vi "InitiateMultiPoint.vi"(8 "error in (no error)":errorcluster, 11 "HP3458aDMM in":refnum<class "HP3458aDMM.lvclass">) -> (0 "error out":errorcluster, 3 "HP3458aDMM out":refnum<class "HP3458aDMM.lvclass">)   [LabVIEW 2014, in "SamplerPlugins.lvlib" / "HP3458aDMM.lvclass"]
uses:
  HP3458aDMM.lvclass
  <instrlib>/Agilent 3458/Agilent 3458.lvlib
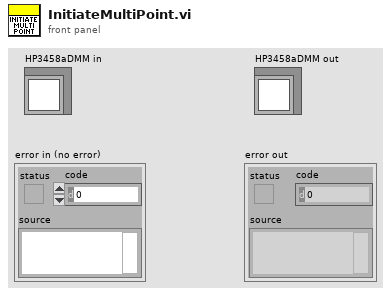
[diagram p1: front panel]
types:
  T1 = typedef "SamplerPlugins.lvlib/SamplerPluginsBase.lvclass/ConfigMultiPointParams.ctl" = cluster{"iTriggerCount":i32, "iSampleCount":i32, "eSampleClock":u16, "dSampleInterval":dbl}
  T2 = typedef "SamplerPlugins.lvlib/SamplerPluginsBase.lvclass/ReadMultiPointParams.ctl" = cluster{"iMaxTimeMilliseconds":i32, "iArraySize":i32}
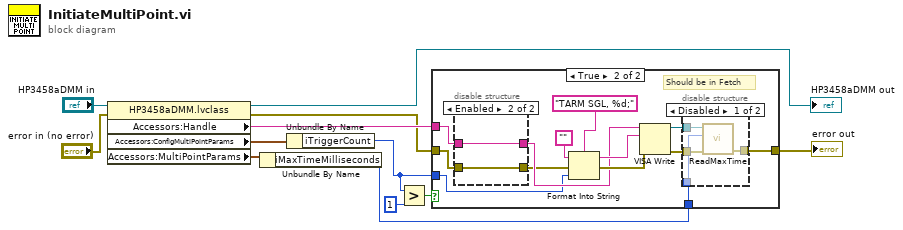
[diagram p0: block diagram]
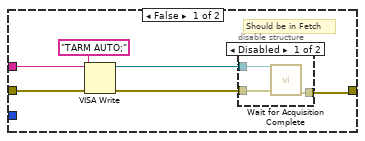
[diagram p2: hidden frame]
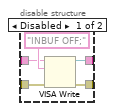
[diagram p5: hidden frame]
diagram:
  n1 = property class="HP3458aDMM.lvclass"(reference="HP3458aDMM in", error in="error in (no error)") -> (reference out=→"HP3458aDMM out":refnum<class "HP3458aDMM.lvclass">, error out=w7:errorcluster, "Accessors:Handle"=w8:string, "Accessors:ConfigMultiPointParams"=w4:T1, "Accessors:MultiPointParams"=w2:T2)
  n2 = Unbundle By Name(w2) -> ("iMaxTimeMilliseconds"=w1:i32)
  n3 = Unbundle By Name(w4) -> ("iTriggerCount"=w3:i32)
  n4 = Greater?(x=w3, y=1) -> (0:w9:bool)
  n5 = case shown="True" w9 {
    tunnel: w8 -> [w17 w30]
    tunnel: w7 -> [w16 w29]
    tunnel: [w13 w24] -> w5
    tunnel: w3 -> [_ w27]
    tunnel: w1 -> [_ w23]
    frame False {
      # "Should be in Fetch"
      n6 = VISA Write(VISA resource name=w17, write buffer="TARM AUTO;", error in (no error)=w16) -> (VISA resource name out=w15:refnum<visa-resource-name>, error out=w14:errorcluster)  [unwired: 1 out]
      n7 = disable-structure shown="Disabled" {
        disable-tunnel: w15 -> [w21 _]
        disable-tunnel: w14 -> [w20 w22]
        disable-tunnel: [w19 w22] -> w13
        frame Disabled {
          n8 = call <instrlib>:"Wait for Acquisition Complete.vi"("error in (no error)"=w20, "VISA resource name"=w21) -> ("error out"=w19:errorcluster)  [unwired: 8 in, 1 out]
        }
        frame Enabled {
        }
      }
    }
    frame True {
      # "Should be in Fetch"
      n9 = disable-structure shown="Enabled" {
        disable-tunnel: [w44 w47] -> w31
        disable-tunnel: w30 -> [w43 w47]
        disable-tunnel: w29 -> [w42 w46]
        disable-tunnel: [w41 w46] -> w28
        frame Disabled {
          n10 = VISA Write(VISA resource name=w43, write buffer="INBUF OFF;", error in (no error)=w42) -> (VISA resource name out=w44:refnum<visa-resource-name>, error out=w41:errorcluster)  [unwired: 1 out]
        }
        frame Enabled {
        }
      }
      n11 = Format Into String(format string="TARM SGL, %d;", initial string="", error in=w28, w27) -> (resulting string=w33:string, error out=w32:errorcluster)
      n12 = VISA Write(VISA resource name=w31, write buffer=w33, error in (no error)=w32) -> (VISA resource name out=w26:refnum<visa-resource-name>, error out=w25:errorcluster)  [unwired: 1 out]
      n13 = disable-structure shown="Disabled" {
        disable-tunnel: w26 -> [w39 _]
        disable-tunnel: w25 -> [w38 w40]
        disable-tunnel: [w37 w40] -> w24
        disable-tunnel: w23 -> [w36 _]
        frame Disabled {
          n14 = call "ReadMaxTime.vi"("error in (no error)"=w38, "iMaxTimeMilliseconds"=w36, "HandleIn"=w39) -> ("error out"=w37:errorcluster)  [unwired: 7 in, 1 out]
        }
        frame Enabled {
        }
      }
    }
  }
  "error out" <- w5
